vi "Do.vi"(8 "error in (no error)":errorcluster, 10 "Actor in":refnum<class "Actor.lvclass">, 11 "PW3390 Actor Msg":refnum<class "PW3390 Actor Msg.lvclass">) -> (0 "error out":errorcluster, 2 "Actor out":refnum<class "Actor.lvclass">)   [LabVIEW 2024, in "PW3390 Actor.lvlib" / "PW3390 Actor Msg.lvclass"]
doc: "<p>(<strong>Filename</strong>: <span class=\"dnl\">Actor Framework.lvlib:Message.lvclass:Do.vi</span>)</p>\n<p>Defines what a message does when it is received by an actor. Generally, a message instructs an actor to invoke one of its methods. By default, this method does nothing. A child class must override it to define behavior.</p>"
uses:
  PW3390 Actor Msg.lvclass
  <vilib>/ActorFramework/Actor/Actor.lvclass
  PW3390/PW3390.lvclass
  C:/Program Files (x86)/National Instruments/LabVIEW 2024/vi.lib/ActorFramework/Actor/Actor.lvclass
  PW3390 Actor Msg.lvclass/PW3390 Actor Msg.ctl
  <vilib>/ActorFramework/Message/Message.lvclass
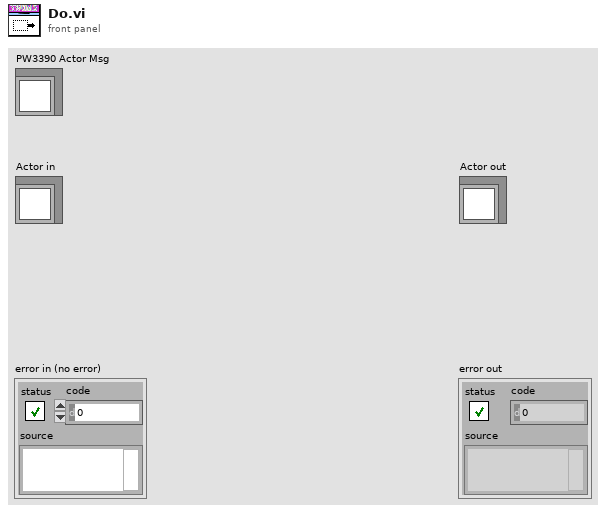
[diagram p1: front panel]
types:
  T1 = typedef "PW3390MsgFunc.ctl" = enum16{"StartQuery", "StopQuery"}
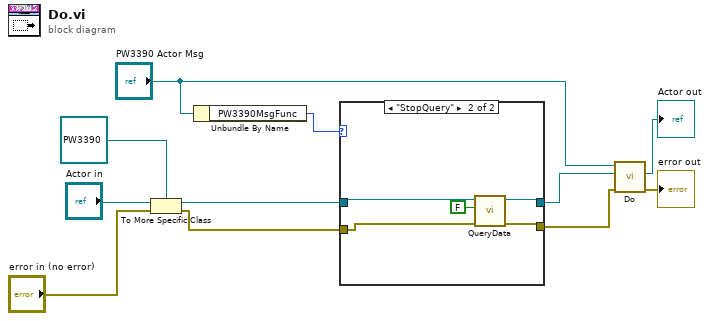
[diagram p0: block diagram]
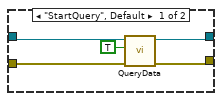
[diagram p2: hidden frame]
diagram:
  n1 = To More Specific Class(target class=refnum<class "PW3390.lvclass"> refnum ("PW3390 Actor.lvlib:PW3390.lvclass"), reference="Actor in", error in="error in (no error)") -> (specific class reference=w4:refnum<class "PW3390.lvclass">, error out=w3:errorcluster)
  n2 = Unbundle By Name("PW3390 Actor Msg") -> ("PW3390MsgFunc"=w5:T1)
  n3 = case shown="\"StopQuery\"" w5 {
    tunnel: w4 -> [w15 w20]
    tunnel: w3 -> [w14 w19]
    tunnel: [w13 w18] -> w2
    tunnel: [w12 w17] -> w1
    frame "StartQuery", Default {
      n4 = call "QueryData.vi"("error in (no error)"=w14, "Query?"=TRUE, "PW3390 in"=w15) -> ("error out"=w12:errorcluster, "PW3390 out"=w13:refnum<class "PW3390.lvclass">)  [unwired: 7 in]
    }
    frame "StopQuery" {
      n5 = call "QueryData.vi"("error in (no error)"=w19, "Query?"=FALSE, "PW3390 in"=w20) -> ("error out"=w17:errorcluster, "PW3390 out"=w18:refnum<class "PW3390.lvclass">)  [unwired: 7 in]
    }
  }
  n6 = call-parent "Do.vi"("error in (no error)"=w1, "Actor in"=w2, "Message"="PW3390 Actor Msg") -> ("error out"=→"error out":errorcluster, "Actor out"=→"Actor out":refnum<class "Actor.lvclass">)  [unwired: 7 in]
